vi "ForwardMotor.vi"(9 "Go":bool, 10 "stop":bool, 11 "RPM":u16) -> ()   [LabVIEW 2019]
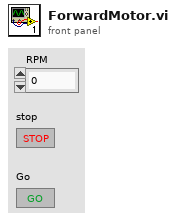
[diagram p1: front panel]
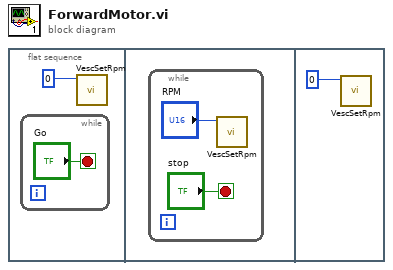
[diagram p0: block diagram]
diagram:
  n1 = flat-sequence {
    frame #0 {
      n2 = while {
        stop <- "Go" stop-if-true
      }
      n3 = call "VescSetRpm.vi"("RPM"=0) -> ()  [unwired: 11 in]
    }
    frame #1 {
      n4 = while {
        stop <- "stop" stop-if-true
        n5 = call "VescSetRpm.vi"("RPM"="RPM") -> ()  [unwired: 11 in]
      }
    }
    frame #2 {
      n6 = call "VescSetRpm.vi"("RPM"=0) -> ()  [unwired: 11 in]
    }
  }
